vi "ex_createorOpenTDMS.vi"(0 "file path in":path, 1 "overwrite_mode_multi":T3(ring), 2 "overwrite_mode":T4(ring), 3 "tdms file in":refnum<k34>, 4 "file dialog?":bool, 5 "error in (no error)":errorcluster, 6 "file params":T1 {"Flags"."time preference" items=["Absolute", "Relative"]; "Flags"."x_columns" items=["None", "One", "Multiple"]; "origin time" format="%<%X\n%x>T"}, 7 "multi_file":bool, 9 "new file?":bool, 11 "Simulate Non-First Call":bool) -> (13 "new file was created":bool, 14 "file path out":path, 15 "dialog was cancelled":bool, 16 "keep loop going":bool, 17 "tdms file out":refnum<k34>, 18 "file params out":T1 {"Flags"."time preference" items=["Absolute", "Relative"]; "Flags"."x_columns" items=["None", "One", "Multiple"]; "origin time" format="%<%X\n%x>T"}, 19 "error out":errorcluster)   [LabVIEW 2020]
uses:
  express output/ExFileWriteBlock.llb/ex_WriteFileParams.ctl
  express input/ExFileReadBlock.llb/ex_ReadFileParams.ctl
  ExFile.llb/ex_FileGlobals.vi
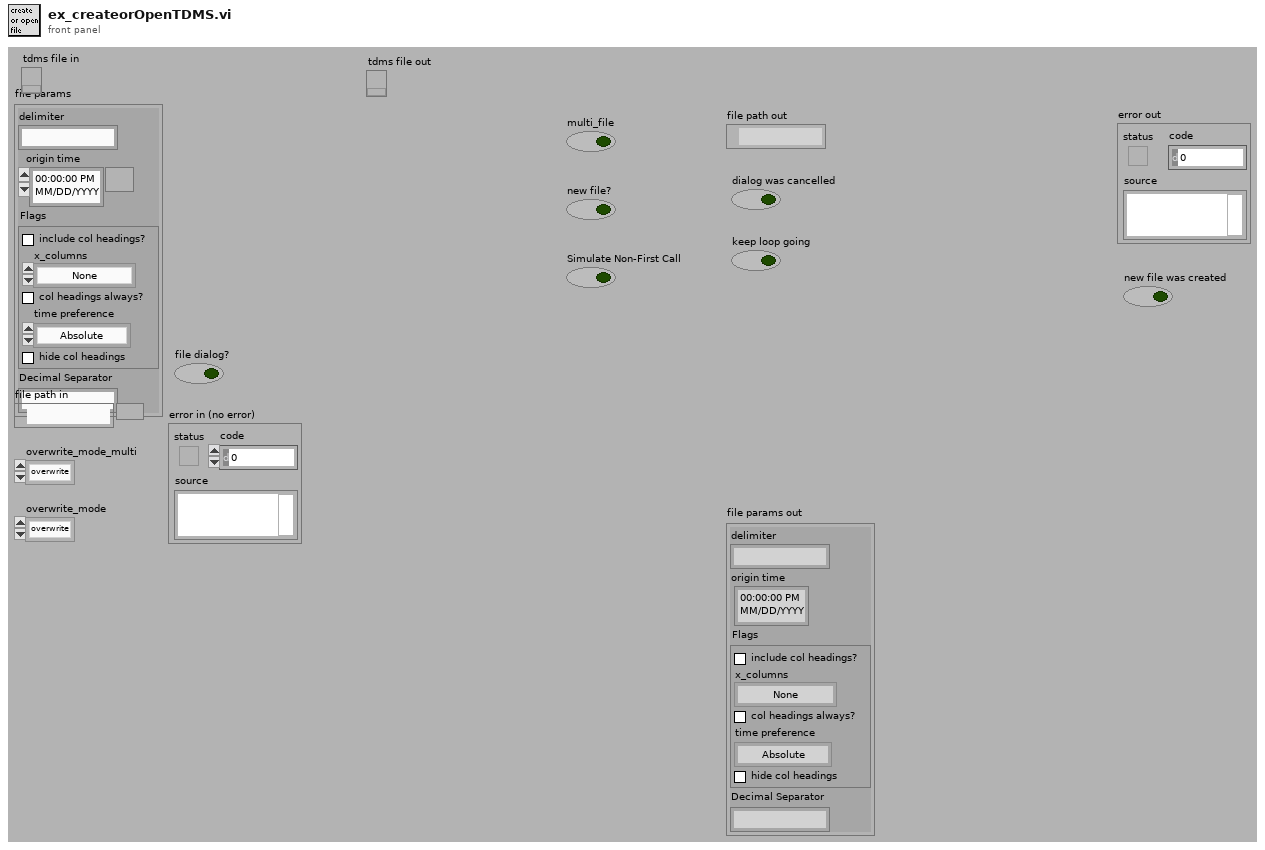
[diagram p1: front panel]
types:
  T1 = typedef "ex_WriteFileParams.ctl" = cluster{"delimiter":string, "origin time":timestamp, "Flags":T2, "Decimal Separator":string}
  T2 = typedef "ex_ReadFileParams.ctl" = cluster{"include col headings?":bool, "x_columns":u16, "col headings always?":bool, "time preference":u16, "hide col headings":bool}
  T3 = enum16{"overwrite", "overwrite & backup", "next avail"}
  T4 = enum16{"overwrite", "overwrite & backup", "append", "next avail"}
  T5 = enum16{"open", "open or create", "create or replace", "create", "open (read-only)"}
  T6 = enum16{"existing file", "new file", "new or existing file", "existing dir", "new dir", "new or existing dir", "existing file (use LLBs)", "new file (use LLBs)", "new or existing file (use LLBs)", "new or existing file or directory (use LLBs)"}
  T7 = cluster{"message":string, "T button name":string, "F button name":string}
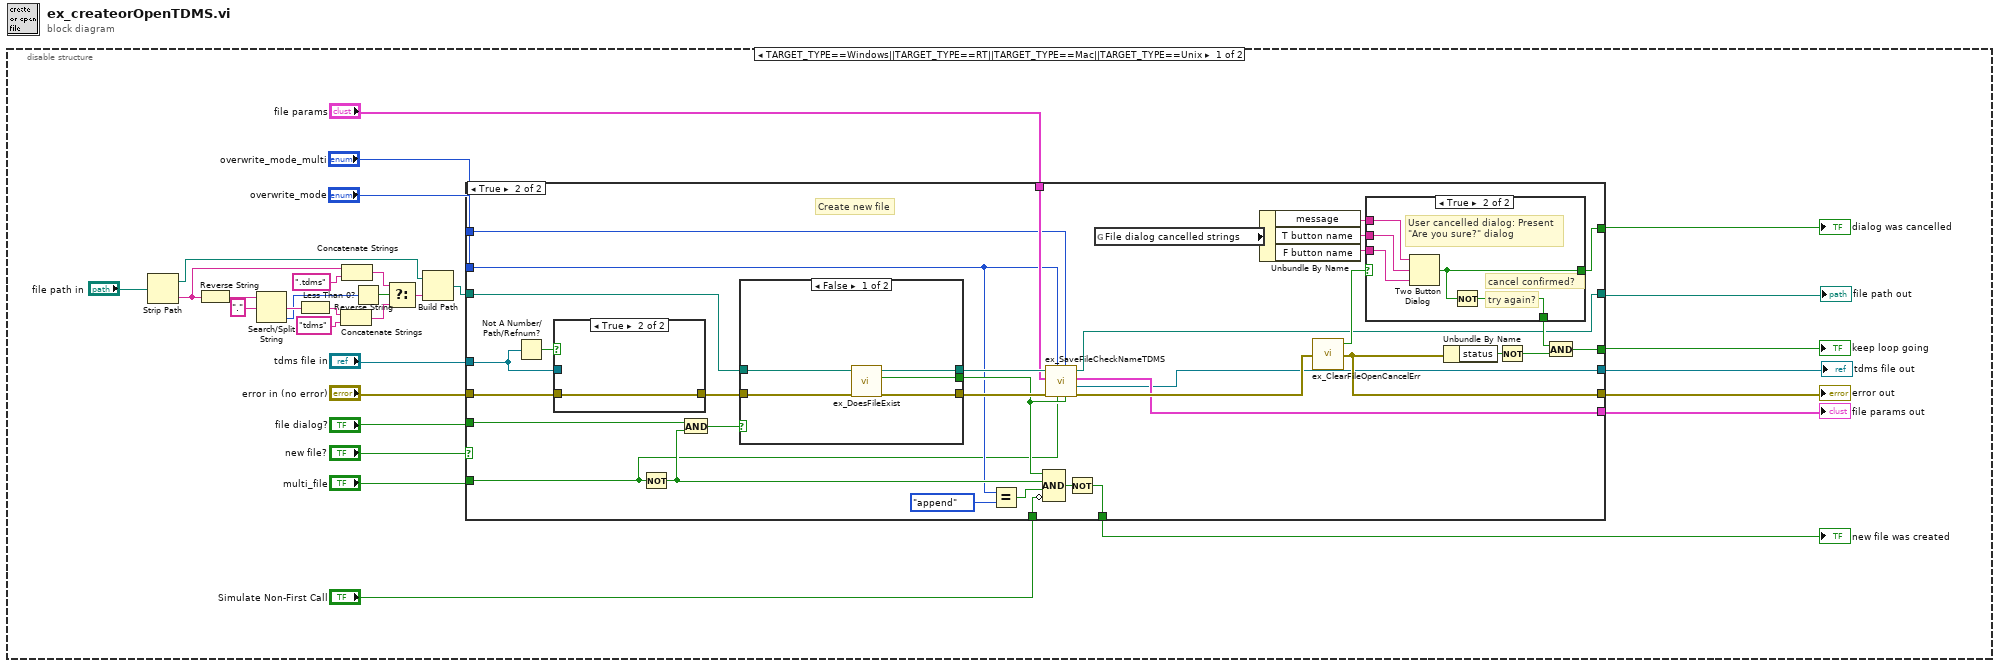
[diagram p0: block diagram]
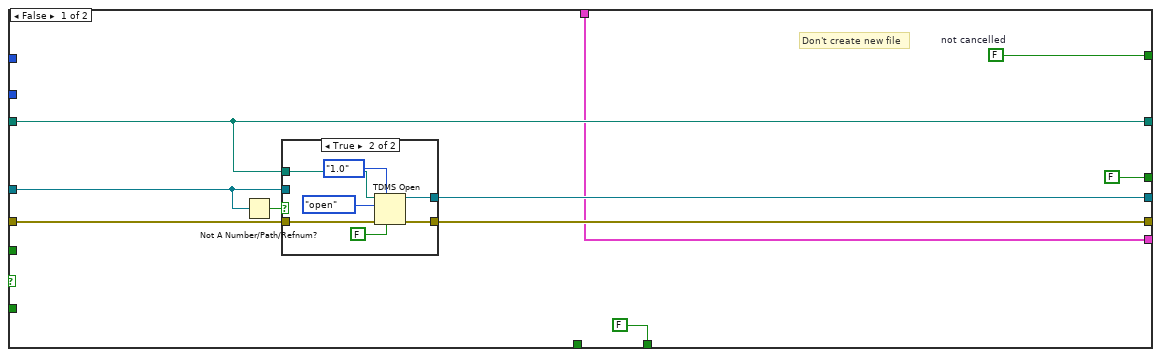
[diagram p2: hidden frame]
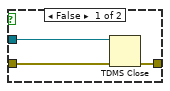
[diagram p4: hidden frame]
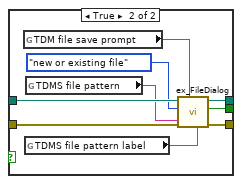
[diagram p6: hidden frame]
diagram:
  n1 = disable-structure shown="TARGET_TYPE==Windows||TARGET_TYPE==RT||TARGET_TYPE==Mac||TARGET_TYPE==Unix" {
    frame condition #0 (active) {
      n2 = Strip Path(path="file path in") -> (stripped path=w2:path, name=w4:string)
      n3 = Reverse String(1:w4) -> (0:w15:string)
      n4 = Search/Split String(string=w15, search string/char (-)=".") -> (match + rest of string=w13:string, offset of match=w10:i32)  [unwired: 2 out]
      n5 = Reverse String(1:w13) -> (0:w11:string)
      n6 = Concatenate Strings(w11, "tdms" ("replace string (\"\")")) -> (w6:string)
      n7 = Concatenate Strings(w4, ".tdms" ("replace string (\"\")")) -> (w7:string)
      n8 = Less Than 0?(x=w10) -> (x < 0?=w9:bool)
      n9 = Select(t=w7, s=w9, f=w6) -> (s? t:f=w3:string)
      n10 = Build Path(base path=w2, name or relative path=w3) -> (appended path=w1:path)
      n11 = case shown="True" "new file?" {
        tunnel: "error in (no error)" -> [w38 w58]
        tunnel: w1 -> [w35 w77]
        tunnel: [w37 w61] -> w28
        tunnel: [w32 w53] -> w29
        tunnel: "Simulate Non-First Call" -> [_ w75]
        tunnel: [w41 w71] -> w26
        tunnel: [FALSE w70] -> w31
        tunnel: [w36 w51] -> w16
        tunnel: "file params" -> [w32 w67]
        tunnel: "multi_file" -> [_ w52]
        tunnel: "file dialog?" -> [_ w66]
        tunnel: "overwrite_mode_multi" -> [_ w65]
        tunnel: "overwrite_mode" -> [_ w64]
        tunnel: [FALSE w59] -> w25
        tunnel: "tdms file in" -> [w33 w55]
        tunnel: [w35 w54] -> w27
        frame False {
          w41 = FALSE  # not cancelled
          # "Don't create new file"
          n12 = Not A Number/Path/Refnum?(number/path/refnum=w33) -> (NaN/Path/Refnum?=w34:bool)
          n13 = case shown="True" w34 {
            tunnel: w38 -> [w43 w50]
            tunnel: [w43 w49] -> w37
            tunnel: [w42 w48] -> w36
            tunnel: w35 -> [_ w47]
            tunnel: w33 -> [w42 _]
            frame False {
            }
            frame True {
              n14 = TDMS Open(6:FALSE ("disable buffering? (T)"), 7:enum16{"1.0", "2.0"}."1.0" ("file format version (2.0)"), 8:w50, 10:T5."open" ("operation"), 11:w47) -> (0:w49:errorcluster, 3:w48:refnum<k34>)  [unwired: 2 in]
            }
          }
        }
        frame True {
          # "Create new file"
          n15 = Not A Number/Path/Refnum?(number/path/refnum=w55) -> (NaN/Path/Refnum?=w56:bool)
          n16 = case shown="True" w56 {
            tunnel: w58 -> [w88 w89]
            tunnel: [w87 w89] -> w57
            tunnel: w55 -> [w86 _]
            frame False {
              n17 = TDMS Close(8:w88, 11:w86) -> (0:w87:errorcluster)  [unwired: 1 out]
            }
            frame True {
            }
          }
          n18 = Not(x=w52) -> (.not. x?=w85:bool)
          n19 = And(x=w66, y=w85) -> (x .and. y?=w84:bool)
          n20 = case shown="False" w84 {
            tunnel: w77 -> [w99 w109]
            tunnel: [w98 w108] -> w73
            tunnel: [w97 w107] -> w74
            tunnel: w57 -> [w100 w106]
            tunnel: [w96 w105] -> w72
            frame False {
              n21 = call "ex_DoesFileExist.vi"("error in"=w100, "file path"=w99) -> ("error out"=w97:errorcluster, "file exists"=w96:bool, "dup file path"=w98:path)  [unwired: 3 out]
            }
            frame True {
              n22 = global read "ex_FileGlobals.vi" "TDM file save prompt"() -> (w103:string)
              n23 = global read "ex_FileGlobals.vi" "TDMS file pattern label"() -> (w102:string)
              n24 = global read "ex_FileGlobals.vi" "TDMS file pattern"() -> (w101:string)
              n25 = call "ex_FileDialog.vi"("pattern label"=w102, "pattern"=w101, "prompt"=w103, "error in (no error)"=w106, "select mode"=T6."new or existing file", "start path"=w109) -> ("error out"=w107:errorcluster, "file exists?"=w105:bool, "selected file path"=w108:path)  [unwired: 3 out]
            }
          }
          n26 = Equal?(x=w64, y=T4."append" ("overwrite_mode")) -> (x = y?=w79:bool)
          n27 = Compound Arithmetic op=AND(w72, w85, w79, invert w75) -> (w78:bool)
          n28 = call "ex_SaveFileCheckNameTDMS.vi"("file exists?"=w72, "overwrite_mode_multi"=w65, "multi_file"=w52, "overwrite_mode"=w64, "error in (no error)"=w74, "file params in"=w67, "file path"=w73) -> ("error out"=w69:errorcluster, "tdms file out"=w51:refnum<k34>, "file params out"=w53:T1, "file path out"=w54:path)  [unwired: 1 out]
          n29 = Not(x=w78) -> (.not. x?=w70:bool)
          n30 = global read "ex_FileGlobals.vi" "File dialog cancelled strings"() -> (w76:T7)
          n31 = Unbundle By Name(w76) -> ("message"=w83:string, "T button name"=w82:string, "F button name"=w81:string)
          n32 = call "ex_ClearFileOpenCancelErr.vi"("error in"=w69) -> ("error out"=w61:errorcluster, "cancelled?"=w68:bool)  [unwired: 3 out]
          n33 = case shown="True" w68 {
            selector: w68 -> [w90 _]
            tunnel: w81 -> [_ w95]
            tunnel: w83 -> [_ w94]
            tunnel: w82 -> [_ w93]
            tunnel: [w90 w92] -> w71
            tunnel: [w90 w91] -> w60
            frame False {
              # "not cancelled"
              # "file dialog not cancelled"
            }
            frame True {
              # "cancel confirmed?"
              # "try again?"
              # "User cancelled dialog: Present\n\"Are you sure?\" dialog"
              n34 = Two Button Dialog(message=w94, 1:w95, 2:w93) -> (T button?=w92:bool)
              n35 = Not(x=w92) -> (.not. x?=w91:bool)
            }
          }
          n36 = Unbundle By Name(w61) -> ("status"=w62:bool)
          n37 = Not(x=w62) -> (.not. x?=w63:bool)
          n38 = And(x=w60, y=w63) -> (x .and. y?=w59:bool)
        }
      }
      "new file was created" <- w31
      "file params out" <- w29
      "error out" <- w28
      "file path out" <- w27
      "dialog was cancelled" <- w26
      "keep loop going" <- w25
      "tdms file out" <- w16
    }
    frame condition #1 {
    }
  }
